vi "PTScanner.get objects.vi"(0 "i ref in":refnum<vi>) -> (16 "objects":string[](array[string]))   [LabVIEW 2014, in "PTScanner.lvlib"]
uses:
  PTScanner.lvlib
  _common/PTUtils/PTUtils.lvlib
  CS_Core/CSSystem/CSSystemLib/CSSystemLib.lvlib
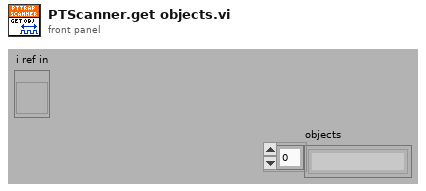
[diagram p1: front panel]
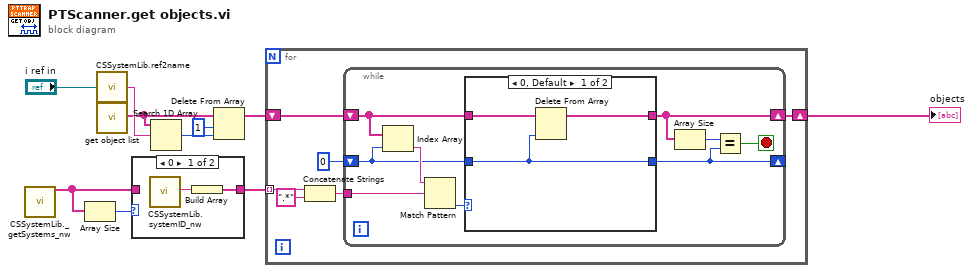
[diagram p0: block diagram]
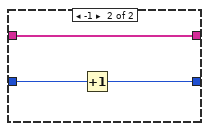
[diagram p2: hidden frame]
diagram:
  n1 = call "CSSystemLib._getSystems_nw.vi"() -> ("CSSystems"=w4:string[])  [unwired: 17 in, 2 out]
  n2 = Array Size(array=w4) -> (size(s)=w5:i32)
  n3 = call "CSSystemLib.ref2name.vi"("obj refnum"="i ref in") -> ("name"=w10:string)
  n4 = call "get object list.vi"() -> ("Objects"=w7:string[])  [unwired: 19 in]
  n5 = case shown="0" w5 {
    tunnel: w4 -> [_ w13]
    tunnel: [w11 w13] -> w1
    frame 0 {
      n6 = call "CSSystemLib.systemID_nw.vi"() -> ("systemID out"=w12:string)  [unwired: 18 in, 1 out]
      n7 = Build Array(w12) -> (w11:string[])
    }
    frame 1, Default {
    }
  }
  n8 = Search 1D Array(1D array=w7, element=w10) -> (index of element=w9:i32)  [unwired: 1 in]
  n9 = Delete From Array(array=w7, length=1, index=w9) -> (array with subset deleted=w6:string[])  [unwired: 1 out]
  n10 = for {
    shift-right: [w15] -> w3
    shift-left: w6 -> [w16]
    tunnel: w1 -> [w14] mode=indexing
    n11 = Concatenate Strings(w14, ".*") -> (w18:string)
    n12 = while {
      shift-right: [w23] -> w15
      shift-left: w16 -> [w26]
      tunnel: w18 -> [w27]
      shift-right: [w21] -> _
      shift-left: 0 -> [w24]
      stop <- w20 stop-if-true
      n13 = Index Array(array=w26, index=w24) -> (element=w25:string)
      n14 = Match Pattern(string=w25, regular expression=w27) -> (offset past match=w28:i32)  [unwired: 1 in, 3 out]
      n15 = case shown="0, Default" w28 {
        tunnel: w26 -> [w31 w34]
        tunnel: [w30 w34] -> w23
        tunnel: w24 -> [w29 w33]
        tunnel: [w29 w32] -> w21
        frame 0, Default {
          n16 = Delete From Array(array=w31, index=w29) -> (array with subset deleted=w30:string[])  [unwired: 1 in, 1 out]
        }
        frame -1 {
          n17 = Increment(x=w33) -> (x+1=w32:i32)
        }
      }
      n18 = Array Size(array=w23) -> (size(s)=w22:i32)
      n19 = Equal?(x=w22, y=w21) -> (x = y?=w20:bool)
    }
  }
  "objects" <- w3
